vi "二型板测试报告存储.vi"(8 "生成报告?":bool, 9 "是否存储到数据库?":bool, 11 "试验时间":timestamp) -> ()   [LabVIEW 2010]
uses:
  <vilib>/Utility/NIReport.llb/NI_report.lvclass
  全局量/试验配置信息.vi
  全局量/自动测试结果.vi
  <vilib>/Utility/NIReport.llb/Append Report Text (str wrap).vi
  <vilib>/addons/_office/word.llb/Word Easy Table (str).vi
  <vilib>/addons/_office/NI_ReportGenerationToolkit.lvlib
panel:
  in  "序号 2":i32
  in  "序号":i32
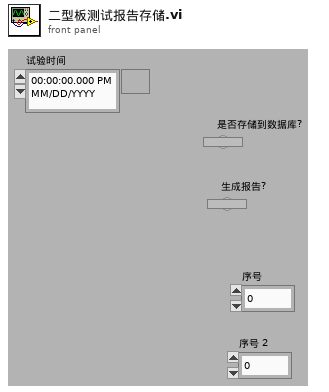
[diagram p1: front panel]
types:
  T1 = enum16{"maximized", "minimized", "normal", "no change"}
  T2 = enum16{"Standard Report", "HTML", "Word", "Excel"}
  T3 = cluster{"position (Excel)":cluster{"row":i32, "column":i32}, "name (Excel)":string, "bookmark (Word)":string}
  T4 = cluster{"报告编号":string, "控制板编号":string, "控制板类型":string, "测试人员":string, "测试地点":string, string, u64, "spreadsheet string":string, "spreadsheet string":string, "spreadsheet string":string, "spreadsheet string":string, "格式字符串":string}
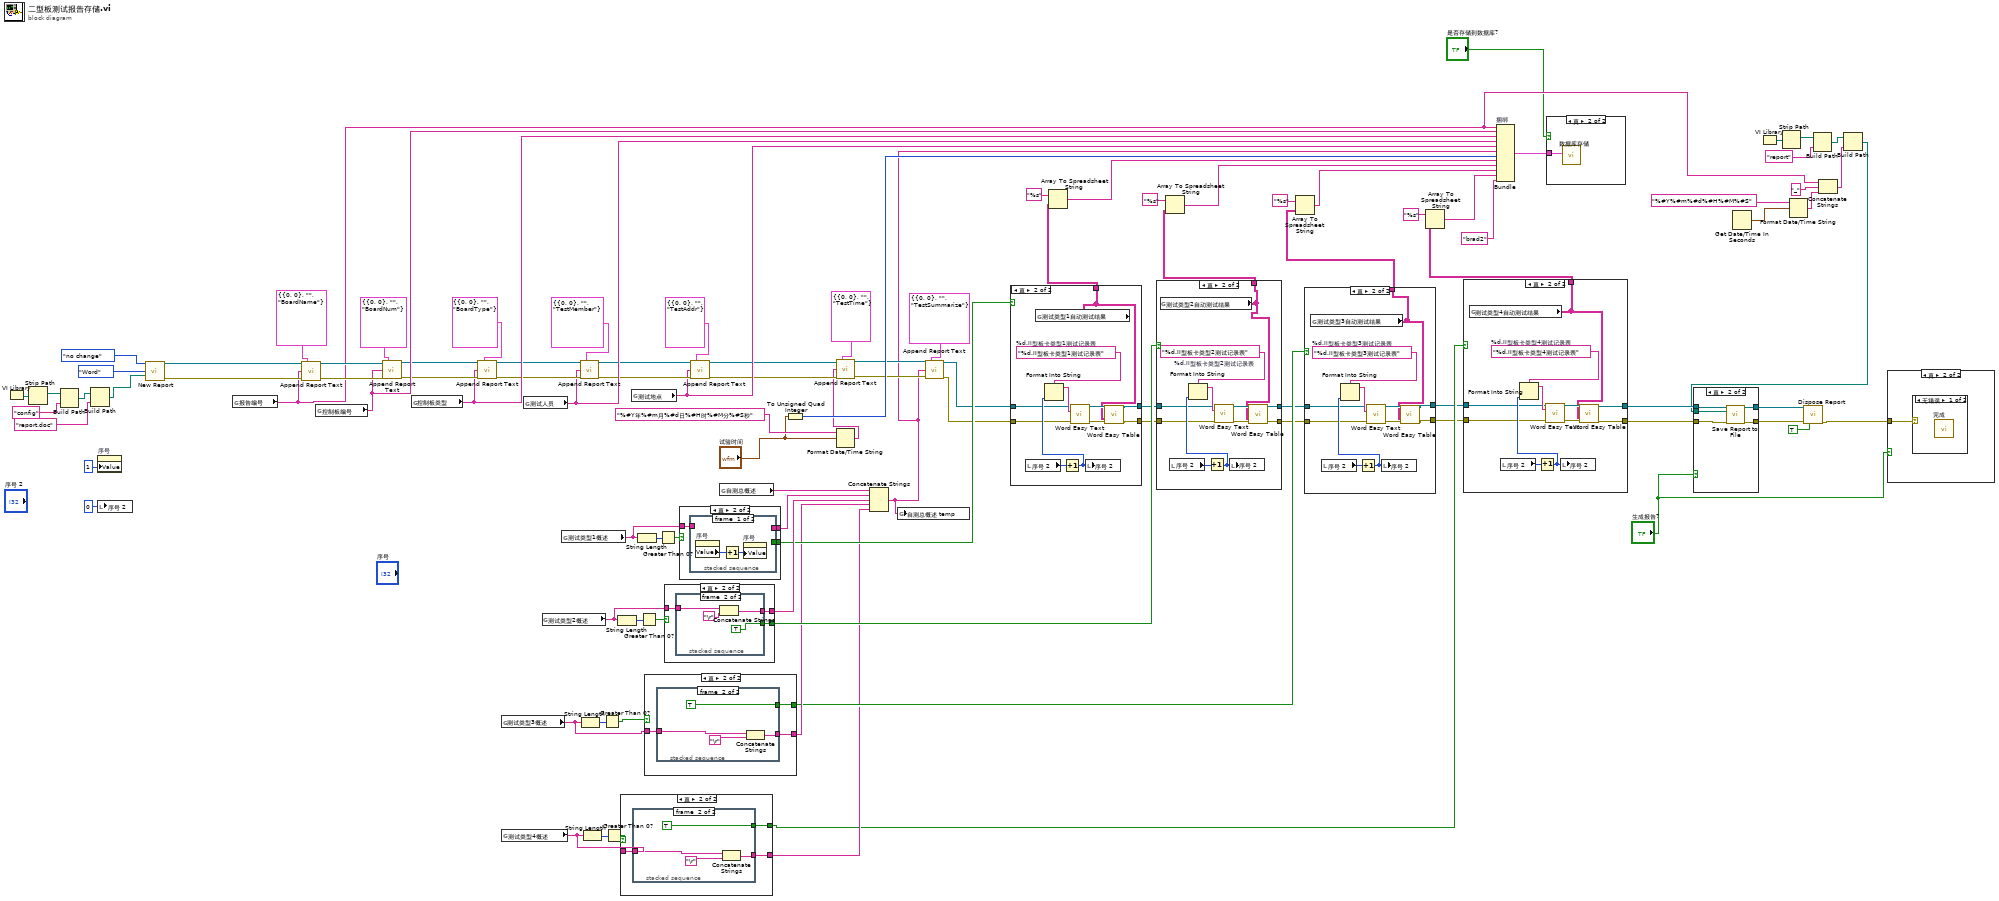
[diagram p0: block diagram]
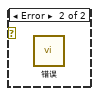
[diagram p3: hidden frame]
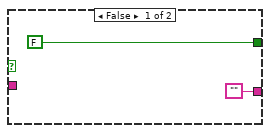
[diagram p6: hidden frame]
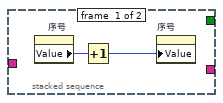
[diagram p7: hidden frame]
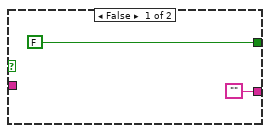
[diagram p8: hidden frame]
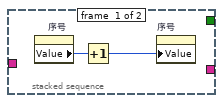
[diagram p9: hidden frame]
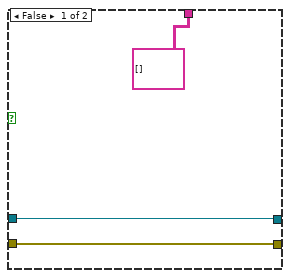
[diagram p10: hidden frame]
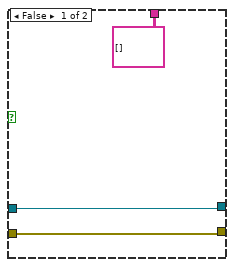
[diagram p11: hidden frame]
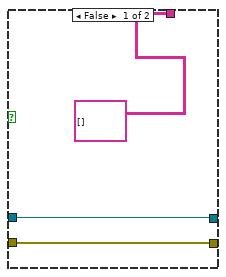
[diagram p12: hidden frame]
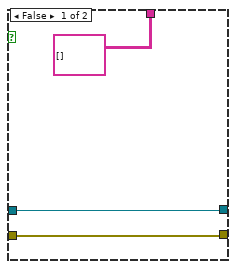
[diagram p13: hidden frame]
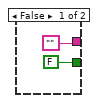
[diagram p14: hidden frame]
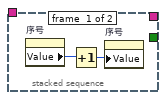
[diagram p15: hidden frame]
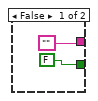
[diagram p16: hidden frame]
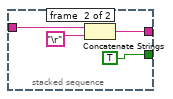
[diagram p17: hidden frame]
diagram:
  n1 = VI Library() -> (path=w63:path)
  n2 = Strip Path(path=w63) -> (stripped path=w60:path)  [unwired: 1 out]
  n3 = Build Path(base path=w60, name or relative path="config") -> (appended path=w62:path)
  n4 = Build Path(base path=w62, name or relative path="report.doc") -> (appended path=w66:path)
  n5 = property on="序号" class="DigNum (严格)"("Value"=1 ("序号")) -> ()  [unwired: 2 in, 2 out]
  n6 = local write "序号 2"(0 ("序号 2")) -> ()
  n7 = call <vilib>:"New Report.vi"("window state (normal)"=T1."no change", "report type"=T2."Word", "template (empty)"=w66) -> ("report out"=w58:refnum<class "NI_report.lvclass">, "error out"=w57:errorcluster)  [unwired: 11 in]
  n8 = global read "试验配置信息.vi" "报告编号"() -> (w4:string)
  n9 = call-poly <vilib>:"Append Report Text.vi"("report in"=w58, "MS Office parameters"=T3 {"position (Excel)"={"row"=0, "column"=0}, "name (Excel)"="", "bookmark (Word)"="BoardName"}, "text"=w4, "error in (no error)"=w57) -> ("report out"=w55:refnum<class "NI_report.lvclass">, "error out"=w54:errorcluster)  [unwired: 8 in, 2 out]
  n10 = global read "试验配置信息.vi" "控制板编号"() -> (w53:string)
  n11 = call-poly <vilib>:"Append Report Text.vi"("report in"=w55, "MS Office parameters"=T3 {"position (Excel)"={"row"=0, "column"=0}, "name (Excel)"="", "bookmark (Word)"="BoardNum"}, "text"=w53, "error in (no error)"=w54) -> ("report out"=w51:refnum<class "NI_report.lvclass">, "error out"=w50:errorcluster)  [unwired: 8 in, 2 out]
  n12 = global read "试验配置信息.vi" "控制板类型"() -> (w49:string)
  n13 = call-poly <vilib>:"Append Report Text.vi"("report in"=w51, "MS Office parameters"=T3 {"position (Excel)"={"row"=0, "column"=0}, "name (Excel)"="", "bookmark (Word)"="BoardType"}, "text"=w49, "error in (no error)"=w50) -> ("report out"=w46:refnum<class "NI_report.lvclass">, "error out"=w45:errorcluster)  [unwired: 8 in, 2 out]
  n14 = global read "自动测试结果.vi" "测试类型3概述"() -> (w73:string)
  n15 = global read "自动测试结果.vi" "测试类型4概述"() -> (w72:string)
  n16 = global read "试验配置信息.vi" "测试人员"() -> (w44:string)
  n17 = global read "自动测试结果.vi" "测试类型2概述"() -> (w100:string)
  n18 = global read "自动测试结果.vi" "测试类型1概述"() -> (w1:string)
  n19 = call-poly <vilib>:"Append Report Text.vi"("report in"=w46, "MS Office parameters"=T3 {"position (Excel)"={"row"=0, "column"=0}, "name (Excel)"="", "bookmark (Word)"="TestMember"}, "text"=w44, "error in (no error)"=w45) -> ("report out"=w42:refnum<class "NI_report.lvclass">, "error out"=w41:errorcluster)  [unwired: 8 in, 2 out]
  n20 = String Length(string=w73) -> (length=w77:i32)
  n21 = String Length(string=w72) -> (length=w70:i32)
  n22 = Greater Than 0?(x=w77) -> (x > 0?=w74:bool)
  n23 = Greater Than 0?(x=w70) -> (x > 0?=w71:bool)
  n24 = String Length(string=w100) -> (length=w98:i32)
  n25 = case shown="真" w71 {
    tunnel: ["" w106] -> w69
    tunnel: w72 -> [_ w107]
    tunnel: [FALSE w105] -> w68
    frame False {
    }
    frame True {
      n26 = stacked-sequence {
        tunnel: w107 -> [_ w113]
        tunnel: [_ w112] -> w106
        tunnel: [_ TRUE] -> w105
        frame #0 {
          n27 = property on="序号" class="DigNum (严格)"() -> ("Value"=w109:i32)  [unwired: 2 in, 2 out]
          n28 = Increment(x=w109) -> (x+1=w108:i32)
          n29 = property on="序号" class="DigNum (严格)"("Value"=w108) -> ()  [unwired: 2 in, 2 out]
        }
        frame #1 {
          n30 = Concatenate Strings(w113, "\r") -> (w112:string)
        }
      }
    }
  }
  n31 = global read "试验配置信息.vi" "测试地点"() -> (w40:string)
  n32 = String Length(string=w1) -> (length=w102:i32)
  n33 = Greater Than 0?(x=w98) -> (x > 0?=w99:bool)
  n34 = case shown="真" w74 {
    tunnel: ["" w117] -> w76
    tunnel: w73 -> [_ w118]
    tunnel: [FALSE w116] -> w75
    frame False {
    }
    frame True {
      n35 = stacked-sequence {
        tunnel: w118 -> [_ w124]
        tunnel: [_ w123] -> w117
        tunnel: [_ TRUE] -> w116
        frame #0 {
          n36 = property on="序号" class="DigNum (严格)"() -> ("Value"=w120:i32)  [unwired: 2 in, 2 out]
          n37 = Increment(x=w120) -> (x+1=w119:i32)
          n38 = property on="序号" class="DigNum (严格)"("Value"=w119) -> ()  [unwired: 2 in, 2 out]
        }
        frame #1 {
          n39 = Concatenate Strings(w124, "\r") -> (w123:string)
        }
      }
    }
  }
  n40 = Greater Than 0?(x=w102) -> (x > 0?=w101:bool)
  n41 = case shown="真" w99 {
    tunnel: w100 -> [_ w129]
    tunnel: ["" w128] -> w95
    tunnel: [FALSE w127] -> w92
    frame False {
    }
    frame True {
      n42 = stacked-sequence {
        tunnel: w129 -> [_ w135]
        tunnel: [_ w133] -> w128
        tunnel: [_ TRUE] -> w127
        frame #0 {
          n43 = property on="序号" class="DigNum (严格)"() -> ("Value"=w131:i32)  [unwired: 2 in, 2 out]
          n44 = Increment(x=w131) -> (x+1=w130:i32)
          n45 = property on="序号" class="DigNum (严格)"("Value"=w130) -> ()  [unwired: 2 in, 2 out]
        }
        frame #1 {
          n46 = Concatenate Strings(w135, "\r") -> (w133:string)
        }
      }
    }
  }
  n47 = case shown="真" w101 {
    tunnel: w1 -> [_ w140]
    tunnel: ["" w139] -> w96
    tunnel: [FALSE w138] -> w93
    frame False {
    }
    frame True {
      n48 = stacked-sequence {
        tunnel: w140 -> [_ w146]
        tunnel: [_ w144] -> w139
        tunnel: [_ TRUE] -> w138
        frame #0 {
          n49 = property on="序号" class="DigNum (严格)"() -> ("Value"=w141:i32)  [unwired: 2 in, 2 out]
          n50 = Increment(x=w141) -> (x+1=w142:i32)
          n51 = property on="序号" class="DigNum (严格)"("Value"=w142) -> ()  [unwired: 2 in, 2 out]
        }
        frame #1 {
          n52 = Concatenate Strings(w146, "\r") -> (w144:string)
        }
      }
    }
  }
  n53 = call-poly <vilib>:"Append Report Text.vi"("report in"=w42, "MS Office parameters"=T3 {"position (Excel)"={"row"=0, "column"=0}, "name (Excel)"="", "bookmark (Word)"="TestAddr"}, "text"=w40, "error in (no error)"=w41) -> ("report out"=w37:refnum<class "NI_report.lvclass">, "error out"=w36:errorcluster)  [unwired: 8 in, 2 out]
  n54 = global read "自动测试结果.vi" "自测总概述"() -> (w97:string)
  n55 = To Unsigned Quad Integer(1:"试验时间") -> (0:w91:u64)
  n56 = Format Date/Time String(time format string (%c)="%#Y年%#m月%#d日%#H时%#M分%#S秒" ("时间格式字符串(%c)"), seconds (now)="试验时间") -> (date/time string=w35:string)  [unwired: 1 in]
  n57 = call-poly <vilib>:"Append Report Text.vi"("report in"=w37, "MS Office parameters"=T3 {"position (Excel)"={"row"=0, "column"=0}, "name (Excel)"="", "bookmark (Word)"="TestTime"}, "text"=w35, "error in (no error)"=w36) -> ("report out"=w33:refnum<class "NI_report.lvclass">, "error out"=w32:errorcluster)  [unwired: 8 in, 2 out]
  n58 = Concatenate Strings(w97, w96, w95, w76, w69) -> (w30:string)
  n59 = global write "自动测试结果.vi" "自测总概述 temp"(w30) -> ()
  n60 = call-poly <vilib>:"Append Report Text.vi"("report in"=w33, "MS Office parameters"=T3 {"position (Excel)"={"row"=0, "column"=0}, "name (Excel)"="", "bookmark (Word)"="TestSummarize"}, "text"=w30, "error in (no error)"=w32) -> ("report out"=w28:refnum<class "NI_report.lvclass">, "error out"=w27:errorcluster)  [unwired: 8 in, 2 out]
  n61 = case shown="真" w93 {
    tunnel: [string[][] [] ("DI自动测试结果") w153] -> w89
    tunnel: w28 -> [w148 w155]
    tunnel: w27 -> [w147 w154]
    tunnel: [w148 w151] -> w26
    tunnel: [w147 w150] -> w25
    frame False {
    }
    frame True {
      w152 = "%d.II型板卡类型1测试记录表"  # %d.II型板卡类型1测试记录表
      n62 = local read "序号 2"() -> (w160:i32)
      n63 = global read "自动测试结果.vi" "测试类型1自动测试结果"() -> (w153:string[][])
      n64 = Increment(x=w160) -> (x+1=w156:i32)
      n65 = Format Into String(format string=w152, w156) -> (resulting string=w159:string)  [unwired: 2 in, 1 out]
      n66 = call <vilib>:"Word Easy Text.vi"("report in"=w155, "text"=w159, "error in (no error)"=w154) -> ("report out"=w157:refnum<class "NI_report.lvclass">, "error out"=w158:errorcluster)  [unwired: 10 in, 1 out]
      n67 = local write "序号 2"(w156) -> ()
      n68 = call-poly <vilib>:"Word Easy Table.vi"("report in"=w157, "data"=w153, "error in (no error)"=w158) -> ("report out"=w151:refnum<class "NI_report.lvclass">, "error out"=w150:errorcluster)  [unwired: 10 in, 1 out]
    }
  }
  n69 = Array To Spreadsheet String(array=w89, 3:"%s" ("格式字符串")) -> (spreadsheet string=w88:string)  [unwired: 1 in]
  n70 = case shown="真" w92 {
    tunnel: [string[][] [] ("DO自动测试结果") w164] -> w86
    tunnel: w26 -> [w163 w169]
    tunnel: w25 -> [w162 w168]
    tunnel: [w163 w166] -> w24
    tunnel: [w162 w165] -> w23
    frame False {
    }
    frame True {
      w167 = "%d.II型板卡类型2测试记录表"  # %d.II型板卡类型2测试记录表
      n71 = global read "自动测试结果.vi" "测试类型2自动测试结果"() -> (w164:string[][])
      n72 = local read "序号 2"() -> (w170:i32)
      n73 = Increment(x=w170) -> (x+1=w174:i32)
      n74 = Format Into String(format string=w167, w174) -> (resulting string=w171:string)  [unwired: 2 in, 1 out]
      n75 = call <vilib>:"Word Easy Text.vi"("report in"=w169, "text"=w171, "error in (no error)"=w168) -> ("report out"=w173:refnum<class "NI_report.lvclass">, "error out"=w172:errorcluster)  [unwired: 10 in, 1 out]
      n76 = local write "序号 2"(w174) -> ()
      n77 = call-poly <vilib>:"Word Easy Table.vi"("report in"=w173, "data"=w164, "error in (no error)"=w172) -> ("report out"=w166:refnum<class "NI_report.lvclass">, "error out"=w165:errorcluster)  [unwired: 10 in, 1 out]
    }
  }
  n78 = Array To Spreadsheet String(array=w86, 3:"%s" ("格式字符串")) -> (spreadsheet string=w85:string)  [unwired: 1 in]
  n79 = case shown="真" w75 {
    tunnel: [string[][] [] ("AI自动测试结果") w180] -> w83
    tunnel: w24 -> [w176 w183]
    tunnel: w23 -> [w175 w182]
    tunnel: [w176 w179] -> w22
    tunnel: [w175 w178] -> w21
    frame False {
    }
    frame True {
      w181 = "%d.II型板卡类型3测试记录表"  # %d.II型板卡类型3测试记录表
      n80 = global read "自动测试结果.vi" "测试类型3自动测试结果"() -> (w180:string[][])
      n81 = local read "序号 2"() -> (w188:i32)
      n82 = Increment(x=w188) -> (x+1=w184:i32)
      n83 = Format Into String(format string=w181, w184) -> (resulting string=w187:string)  [unwired: 2 in, 1 out]
      n84 = call <vilib>:"Word Easy Text.vi"("report in"=w183, "text"=w187, "error in (no error)"=w182) -> ("report out"=w185:refnum<class "NI_report.lvclass">, "error out"=w186:errorcluster)  [unwired: 10 in, 1 out]
      n85 = local write "序号 2"(w184) -> ()
      n86 = call-poly <vilib>:"Word Easy Table.vi"("report in"=w185, "data"=w180, "error in (no error)"=w186) -> ("report out"=w179:refnum<class "NI_report.lvclass">, "error out"=w178:errorcluster)  [unwired: 10 in, 1 out]
    }
  }
  n87 = Array To Spreadsheet String(array=w83, 3:"%s" ("格式字符串")) -> (spreadsheet string=w82:string)  [unwired: 1 in]
  n88 = case shown="真" w68 {
    tunnel: [string[][] [] ("总线通信自测结果") w194] -> w80
    tunnel: w22 -> [w190 w197]
    tunnel: w21 -> [w189 w196]
    tunnel: [w190 w193] -> w7
    tunnel: [w189 w192] -> w6
    frame False {
    }
    frame True {
      w195 = "%d.II型板卡类型4测试记录表"  # %d.II型板卡类型4测试记录表
      n89 = global read "自动测试结果.vi" "测试类型4自动测试结果"() -> (w194:string[][])
      n90 = local read "序号 2"() -> (w198:i32)
      n91 = Increment(x=w198) -> (x+1=w202:i32)
      n92 = Format Into String(format string=w195, w202) -> (resulting string=w199:string)  [unwired: 2 in, 1 out]
      n93 = call <vilib>:"Word Easy Text.vi"("report in"=w197, "text"=w199, "error in (no error)"=w196) -> ("report out"=w201:refnum<class "NI_report.lvclass">, "error out"=w200:errorcluster)  [unwired: 10 in, 1 out]
      n94 = local write "序号 2"(w202) -> ()
      n95 = call-poly <vilib>:"Word Easy Table.vi"("report in"=w201, "data"=w194, "error in (no error)"=w200) -> ("report out"=w193:refnum<class "NI_report.lvclass">, "error out"=w192:errorcluster)  [unwired: 10 in, 1 out]
    }
  }
  n96 = Array To Spreadsheet String(array=w80, 3:"%s" ("格式字符串")) -> (spreadsheet string=w79:string)  [unwired: 1 in]
  n97 = Bundle "捆绑"("报告编号"=w4, "控制板编号"=w53, "控制板类型"=w49, "测试人员"=w44, "测试地点"=w40, w30, w91, "spreadsheet string"=w88, "spreadsheet string"=w85, "spreadsheet string"=w82, "spreadsheet string"=w79, "格式字符串"="brad2") -> (w78:T4)  [unwired: 1 in]
  n98 = case shown="真" "是否存储到数据库?" {
    tunnel: w78 -> [_ w203]
    frame False {
    }
    frame True {
      n99 = call "数据库存储.vi"("输出簇 2"=w203) -> ()  [unwired: 10 in]
    }
  }
  n100 = Get Date/Time In Seconds() -> (seconds since 1Jan1904=w16:timestamp)
  n101 = VI Library() -> (path=w17:path)
  n102 = Strip Path(path=w17) -> (stripped path=w20:path)  [unwired: 1 out]
  n103 = Format Date/Time String(time format string (%c)="%#Y%#m%#d%#H%#M%#S" ("时间格式字符串(%c)"), seconds (now)=w16) -> (date/time string=w14:string)  [unwired: 1 in]
  n104 = Build Path(base path=w20, name or relative path="report") -> (appended path=w18:path)
  n105 = Concatenate Strings(w4, "_", w14) -> (w12:string)
  n106 = Build Path(base path=w18, name or relative path=w12) -> (appended path=w5:path)
  n107 = case shown="真" "生成报告?" {
    tunnel: w7 -> [w205 w210]
    tunnel: w6 -> [w204 w209]
    tunnel: [w205 w208] -> w10
    tunnel: [w204 w207] -> w9
    tunnel: w5 -> [_ w206]
    frame False {
    }
    frame True {
      n108 = call-dynamic "Save Report to File.vi"("report in"=w210, "report file path"=w206, "error in (no error)"=w209) -> ("report out"=w208:refnum<class "NI_report.lvclass">, "error out"=w207:errorcluster)  [unwired: 11 in]
    }
  }
  n109 = call-dynamic "Dispose Report.vi"("report in"=w10, "error in (no error)"=w9, "close report? (T)"=TRUE) -> ("error out"=w8:errorcluster)  [unwired: 12 in]
  n110 = case shown="真" "生成报告?" {
    tunnel: w8 -> [_ w211]
    frame False {
    }
    frame True {
      n111 = case shown="无错误" w211 {
        frame No Error {
          n112 = call "完成"() -> ()  [unwired: 10 in, 2 out]
        }
        frame Error {
          n113 = call "错误"() -> ()  [unwired: 10 in, 2 out]
        }
      }
    }
  }
